vi "记录Process.vi"(8 "error in (no error)":errorcluster caption="错误输入（无错误）", 9 "采集通道":string, 11 "记录":string) -> (0 "error out":errorcluster)   [LabVIEW 2015]
panel:
  out "path":path
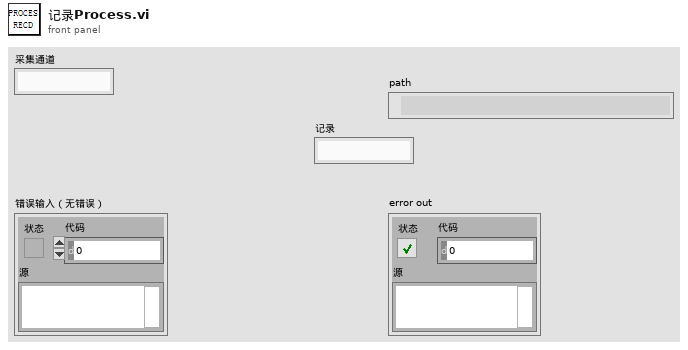
[diagram p1: front panel]
types:
  T1 = enum16{"open", "replace", "create", "open or create", "replace or create", "replace or create with confirmation"}
  T2 = typedef "LVDateTimeRec.ctl" = cluster{"秒数的小数部分":dbl, "秒":i32, "分":i32, "时":i32, "日":i32, "月":i32, "年":i32, "天数（周）":i32, "天数（年）":i32, "DST":i32}
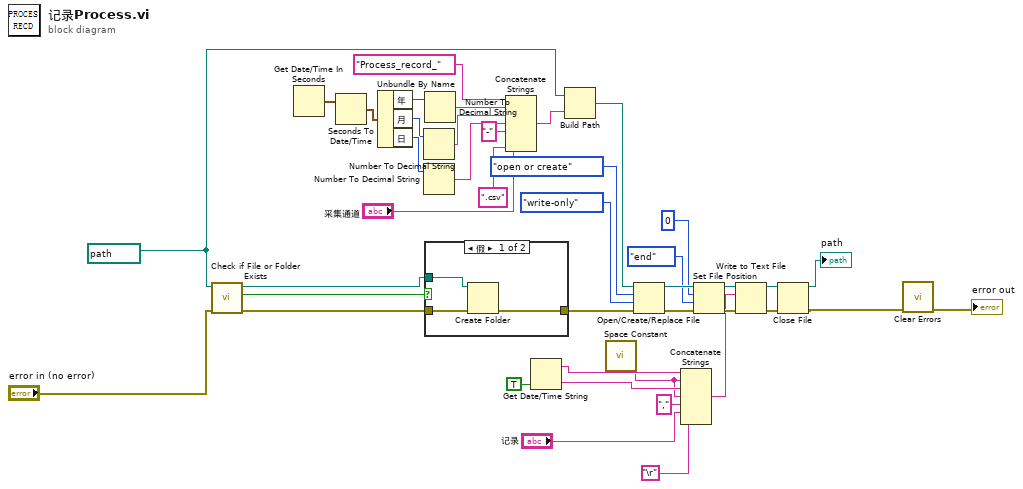
[diagram p0: block diagram]
diagram:
  w11 = path "E:/数据" ("基路径")
  n1 = call <vilib>:"Check if File or Folder Exists.vi"("error in (no error)"="error in (no error)", "path"=w11) -> ("error out"=w15:errorcluster, "file or folder exists?"=w17:bool, "dup path"=w16:path)  [unwired: 7 out]
  n2 = Get Date/Time In Seconds() -> (seconds since 1Jan1904=w18:timestamp)
  n3 = Seconds To Date/Time(time stamp (now)=w18) -> (date time rec=w19:T2)  [unwired: 1 in]
  n4 = Unbundle By Name(w19) -> ("年"=w21:i32, "月"=w20:i32, "日"=w40:i32)
  n5 = Number To Decimal String(number=w20) -> (decimal integer string=w23:string)  [unwired: 1 in]
  n6 = Number To Decimal String(number=w40) -> (decimal integer string=w41:string)  [unwired: 1 in]
  n7 = Number To Decimal String(number=w21) -> (decimal integer string=w22:string)  [unwired: 1 in]
  n8 = case shown="假" w17 {
    tunnel: w16 -> [w44 _]
    tunnel: w15 -> [w43 w45]
    tunnel: [w42 w45] -> w35
    frame False {
      n9 = Create Folder(path (use dialog)=w44, error in=w43) -> (error out=w42:errorcluster)  [unwired: 3 out]
    }
    frame True {
    }
  }
  n10 = Concatenate Strings("Process_record_" ("字符串"), w22, w23, w41, "-" ("字符串"), "采集通道", ".csv" ("字符串")) -> (w24:string)
  n11 = Get Date/Time String(want seconds? (F)=TRUE ("需要秒？(F)")) -> (date string=w9:string, time string=w7:string)  [unwired: 2 in]
  n12 = Build Path(base path=w11, name or relative path=w24) -> (appended path=w38:path)
  n13 = call <vilib>:"Space Constant.vi"() -> ("String"=w6:string)
  n14 = Open/Create/Replace File(file path (use dialog)=w38, error in=w35, operation (0:open)=T1."open or create" ("操作(0:open)"), access (0:read/write)=enum16{"read/write", "read-only", "write-only"}."write-only" ("权限(0:read/write)")) -> (refnum out=w34:refnum<file>, error out=w33:errorcluster)  [unwired: 2 in, 1 out]
  n15 = Concatenate Strings(w9, w6, w7, w6, "," ("字符串"), "记录", "\r") -> (w10:string)
  n16 = Set File Position(offset (in bytes) (0)=i64 0 ("偏移量（字节）（0）"), refnum=w34, from (0:start)=enum16{"start", "end", "current"}."end" ("自（0:起始）"), error in=w33) -> (refnum out=w26:refnum<file>, error out=w29:errorcluster)
  n17 = Write to Text File(file (use dialog)=w26, text=w10, error in=w29) -> (refnum out=w31:refnum<file>, error out=w30:errorcluster)  [unwired: 1 in, 1 out]
  n18 = Close File(refnum=w31, error in=w30) -> (path=→"path":path, error out=w14:errorcluster)
  n19 = call <vilib>:"Clear Errors.vi"("error in (no error)"=w14) -> ("error out"=→"error out":errorcluster)  [unwired: 5 in, 1 out]
